vi "FTW-STR-Split.vi"(5 "Delimited String":string, 7 "Delimiter":string=",") -> (6 "Array of Strings":string[](array[string]))   [LabVIEW 2013]
uses:
  <vilib>/regexp/Match Regular Expression.xnode
panel:
  # "Inputs"
  # "Outputs"
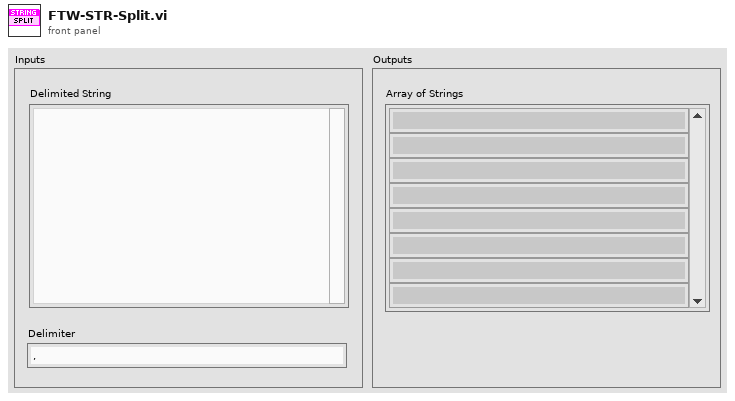
[diagram p1: front panel]
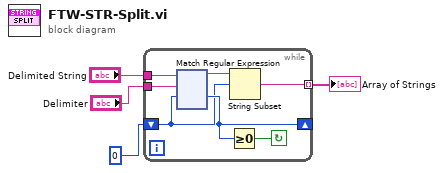
[diagram p0: block diagram]
diagram:
  n1 = while {
    tunnel: "Delimiter" -> [w11]
    tunnel: "Delimited String" -> [w10]
    shift-right: [w9] -> _
    shift-left: 0 ("offset past match") -> [w8]
    tunnel: [w6] -> w1 mode=indexing
    stop <- w5 continue-if-true
    n2 = xnode "Match Regular Expression"("input string"=w10, "regular expression"=w11, "offset (0)"=w8) -> ("before match"=w7:string, "offset past match"=w9:i32)  [unwired: 3 in, 3 out]
    n3 = Greater Or Equal To 0?(x=w9) -> (x >= 0?=w5:bool)
    n4 = String Subset(string=w7, offset (0)=w8) -> (substring=w6:string)  [unwired: 1 in]
  }
  "Array of Strings" <- w1
